vi "move_motor_system.vi"(8 "error in (no error)":errorcluster caption="错误输入（无错误）", 9 "init? (T)":bool=TRUE, 10 "move info array":T1[](array[typedef]), 11 "MotorSystem 输入":refnum<class "MotorSystem.lvclass">) -> (0 "error out":errorcluster caption="错误输出", 3 "MotorSystem 输出":refnum<class "MotorSystem.lvclass">)   [LabVIEW 2016, in "MotionControl_UFO_3DOF.lvlib" / "MotorSystem.lvclass"]
uses:
  <userlib>/MotionControl_UFO_3DOF/MotorSystem/MotorSystem.lvclass
  <userlib>/MotionControl_UFO_3DOF/MotorSystem/MoveInfoCluster.ctl
  <userlib>/MotionControl_UFO_3DOF/MotorSystem/MotorSystem.lvclass/MotorSystem.ctl
  <userlib>/MotionControl_UFO_3DOF/OneMotion/OneMotion.lvclass
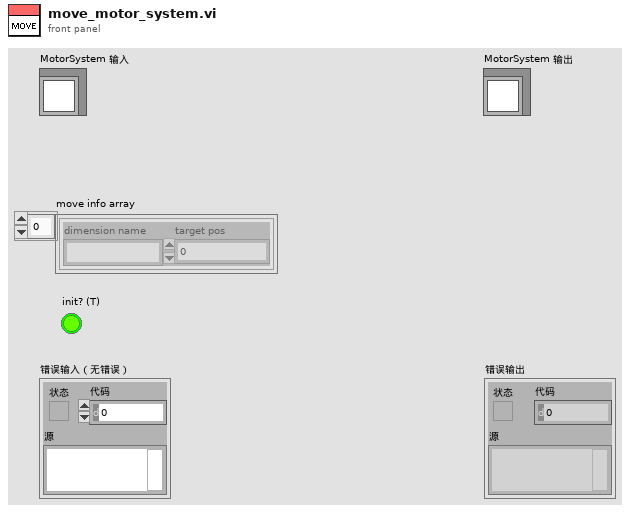
[diagram p1: front panel]
types:
  T1 = typedef "MotionControl_UFO_3DOF.lvlib/MotorSystem.lvclass/MoveInfoCluster.ctl" = cluster{"dimension name":string, "target pos":dbl}
  T2 = typedef "MotionControl_UFO_3DOF.lvlib/MotorSystem.lvclass/MotionCluster.ctl" = cluster{"OneMotion.lvclass":refnum<class "OneMotion.lvclass">, "connected?":bool, "default enabled?":bool, "enabled?":bool}
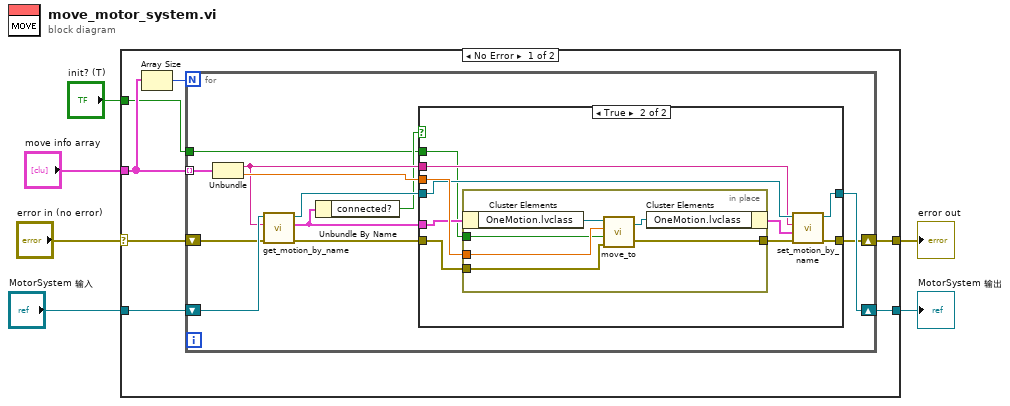
[diagram p0: block diagram]
diagram:
  n1 = case shown="No Error" "error in (no error)" {
    selector: "error in (no error)" -> [w9 w45]
    tunnel: [w8 w45] -> w5
    tunnel: [w10 w44] -> w3
    tunnel: "MotorSystem 输入" -> [w11 w44]
    tunnel: "move info array" -> [w12 _]
    tunnel: "init? (T)" -> [w7 _]
    frame No Error {
      n2 = Array Size(array=w12) -> (size(s)=w13:i32)
      n3 = for {
        N: w13 -> [_]
        tunnel: w12 -> [w25] mode=indexing
        shift-right: [w20] -> w10
        shift-left: w11 -> [w24]
        shift-right: [w17] -> w8
        shift-left: w9 -> [w19]
        tunnel: w7 -> [w14]
        n4 = Unbundle(w25) -> ("dimension name"=w21:string, "target pos"=w23:dbl)
        n5 = call <userlib>:"get_motion_by_name.vi"("error in (no error)"=w19, "name"=w21, "MotorSystem in"=w24) -> ("error out"=w18:errorcluster, "motion cluster"=w16:T2, "MotorSystem out"=w22:refnum<class "MotorSystem.lvclass">)  [unwired: 6 in]
        n6 = Unbundle By Name(w16) -> ("connected?"=w15:bool)
        n7 = case shown="True" w15 {
          tunnel: w23 -> [_ w37]
          tunnel: w22 -> [w27 w36]
          tunnel: w21 -> [_ w35]
          tunnel: [w27 w33] -> w20
          tunnel: w18 -> [w26 w32]
          tunnel: [w26 w30] -> w17
          tunnel: w16 -> [_ w29]
          tunnel: w14 -> [_ w28]
          frame False {
          }
          frame True {
            n8 = in-place {
              in-place-border: w37 -> [w42]
              in-place-border: w32 -> [w40]
              in-place-border: [w39] -> w31
              in-place-border: w28 -> [w38]
              n9 = in-place-cluster #1(w29) -> ("OneMotion.lvclass"=w43:refnum<class "OneMotion.lvclass">)
              n10 = call <userlib>:"move_to.vi"("error in (no error)"=w40, "init? (T)"=w38, "target pos"=w42, "OneMotion 输入"=w43) -> ("error out"=w39:errorcluster, "OneMotion 输出"=w41:refnum<class "OneMotion.lvclass">)
              n11 = in-place-cluster #1("OneMotion.lvclass"=w41) -> (w34:T2)
            }
            n12 = call <userlib>:"set_motion_by_name.vi"("error in (no error)"=w31, "簇"=w34, "name"=w35, "MotorSystem输入"=w36) -> ("error out"=w30:errorcluster, "MotorSystem输出"=w33:refnum<class "MotorSystem.lvclass">)  [unwired: 6 in]
          }
        }
      }
    }
    frame Error {
    }
  }
  "error out" <- w5
  "MotorSystem 输出" <- w3
